vi "class_data.vi"() -> ()   [LabVIEW 2010, in "GenericDisplay.lvclass"]
uses:
  GenericDisplay.lvclass
panel:
  in  "latest instance":refnum<class "GenericDisplay.lvclass">
  in  "trigger queue name":string="display trigger queue"
  in  "locked by":string="DL090216Display_statechart.lvsc:Diagram.vi:Instance:2 > DL090216Display_statechart.lvsc:CompanionDiagram.vi:Instance:20:Instance:EnterGraphCore.vi:2 > DL090216Display_statechart.lvsc:CompanionDiagram.vi:Instance:20:Instance:SC Main.vi:1 > DL090216Display.lvclass:run.vi > main.viDL090216Display_statechart - initialising state"
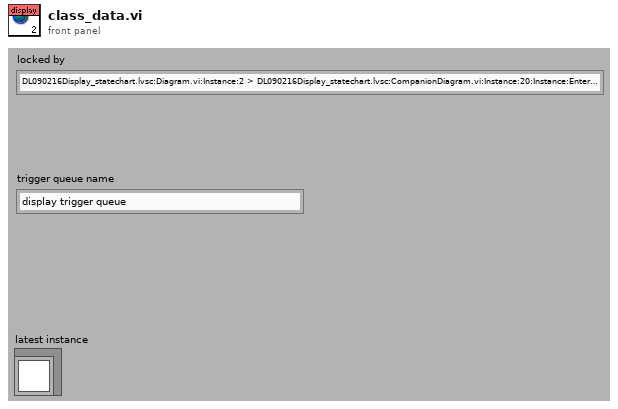
[diagram p1: front panel]
diagram:
